vi "InitWriter.vi"(10 "String":string, 11 "writer name in":string) -> (0 "error out":errorcluster, 3 "writer endpoint":refnum<k21>)   [LabVIEW 2018]
uses:
  RT/Queue/RTMainQueueElements.ctl
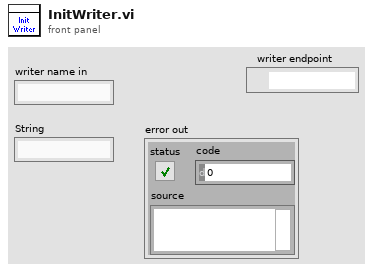
[diagram p1: front panel]
types:
  T1 = typedef "RTMainQueueElements.ctl" = enum16{"RTMain_InitQ", "RTMain_InitSW", "RTMain_InitCtrls", "RTMain_ReInitHW", "RTMain_FromStream", "RTMain_StrtHWLp", "RTMain_UpdtHWClstr", "RTMain_Start", "RTMain_Stop", "RTMain_Error", "RTMain_Config", "RTMain_Exit"}
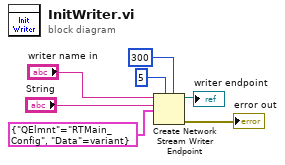
[diagram p0: block diagram]
diagram:
  n1 = Create Network Stream Writer Endpoint(5:300 ("timeout in ms (-1)"), 7:5 ("writer buffer size"), 9:cluster{"QElmnt":T1, "Data":variant} {"QElmnt"=enum."RTMain_Config", "Data"=variant} ("Cluster"), 10:"String", 11:"writer name in") -> (0:→"error out":errorcluster, 3:→"writer endpoint":refnum<k21>)  [unwired: 2 in]
